vi "Set XY Graph Point Style.vi"(8 "Point Style":u8, 9 "Number":i32=1, 10 "Active Plot Start":i32, 11 "XY Graph Reference In":refnum<vi>) -> (3 "XY Graph Reference Out":refnum<vi>)   [LabVIEW 2024]
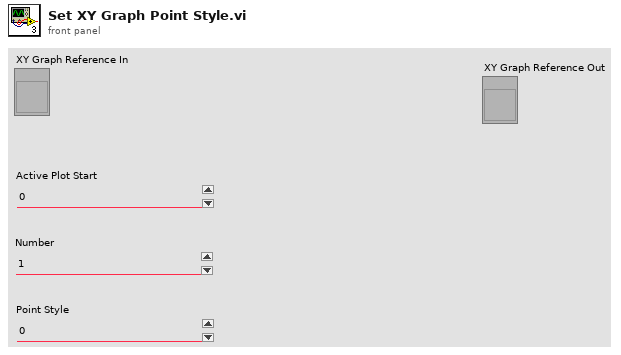
[diagram p1: front panel]
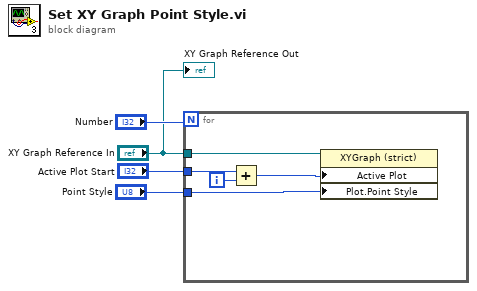
[diagram p0: block diagram]
diagram:
  n1 = for {
    N: "Number" -> [_]
    tunnel: "XY Graph Reference In" -> [w9]
    tunnel: "Active Plot Start" -> [w8]
    tunnel: "Point Style" -> [w5]
    i -> [w7]
    n2 = Add(x=w8, y=w7) -> (x+y=w6:i32)
    n3 = property class="XYGraph (strict)"(reference=w9, "Active Plot"=w6, "Plot.Point Style"=w5) -> ()  [unwired: 1 in, 2 out]
  }
  "XY Graph Reference Out" <- "XY Graph Reference In"
